vi "sweep over IDs.vi"() -> ()   [LabVIEW 2021, in "uCanDriver.lvlib" / "uCAN.lvclass"]
uses:
  uCAN.lvclass
  typedefs/bitrates.ctl
  typedefs/frame.ctl
panel:
  out "current ID":u32 format="%.0x"
  in  "Delay":i16
  in  "Stop":u32 format="%.0x"
  in  "Start":u32 format="%.0x"
  in  "Trace length":u64=100
  out "Table Control":string[][](table)
  in  "New Frame":T1 {"Data" format="%.0x"}
  in  "Bitrates":T2=enum."500 kbit/s"
  in  "COM port":refnum<visa-resource-name>="COM9"
  in  "stop":bool
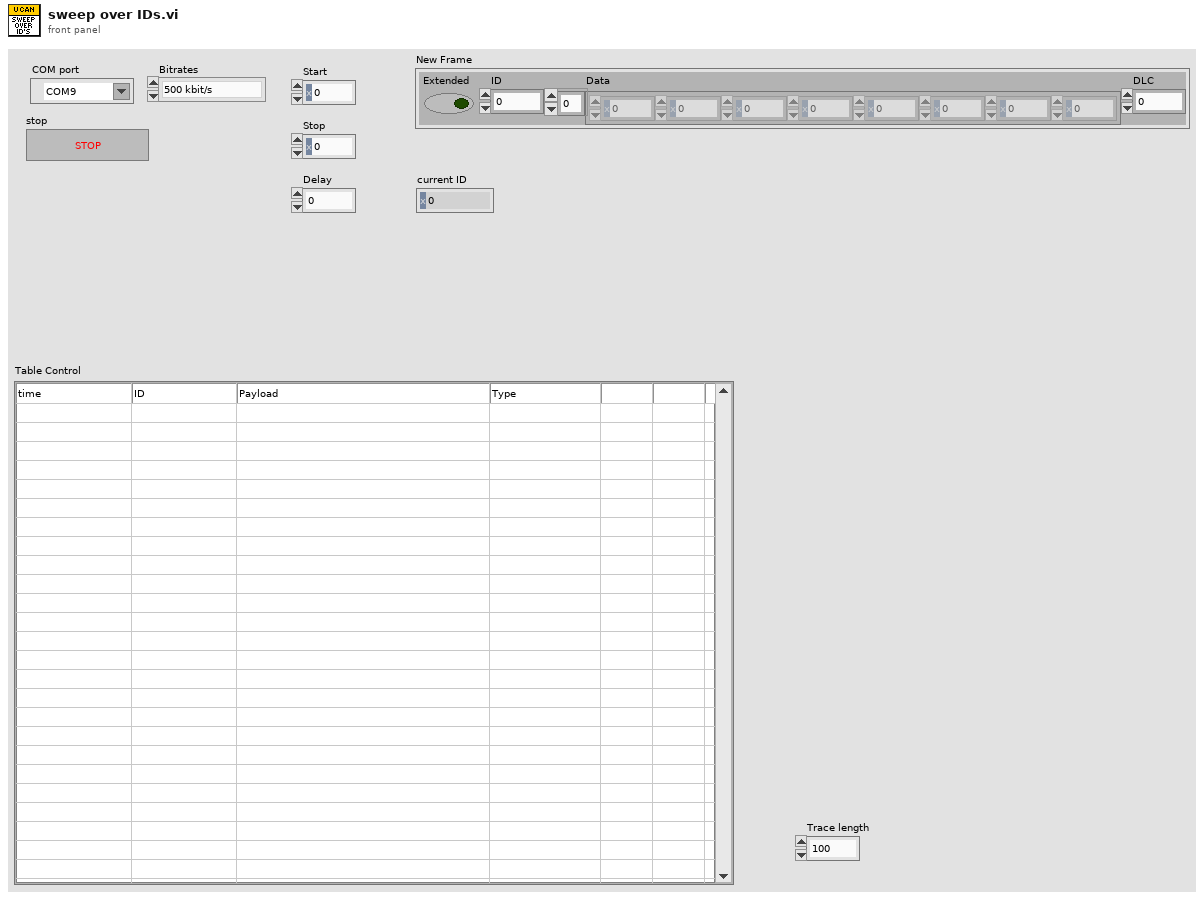
[diagram p1: front panel]
types:
  T1 = typedef "uCanDriver.lvlib/uCAN.lvclass/frame.ctl" = cluster{"Extended":bool, "ID":u32, "Data":u8[], "DLC":u8}
  T2 = typedef "uCanDriver.lvlib/uCAN.lvclass/bitrates.ctl" = enum16{"100 kbit/s", "125 kbit/s", "250 kbit/s", "500 kbit/s", "800 kbit/s", "1 Mbit/s"}
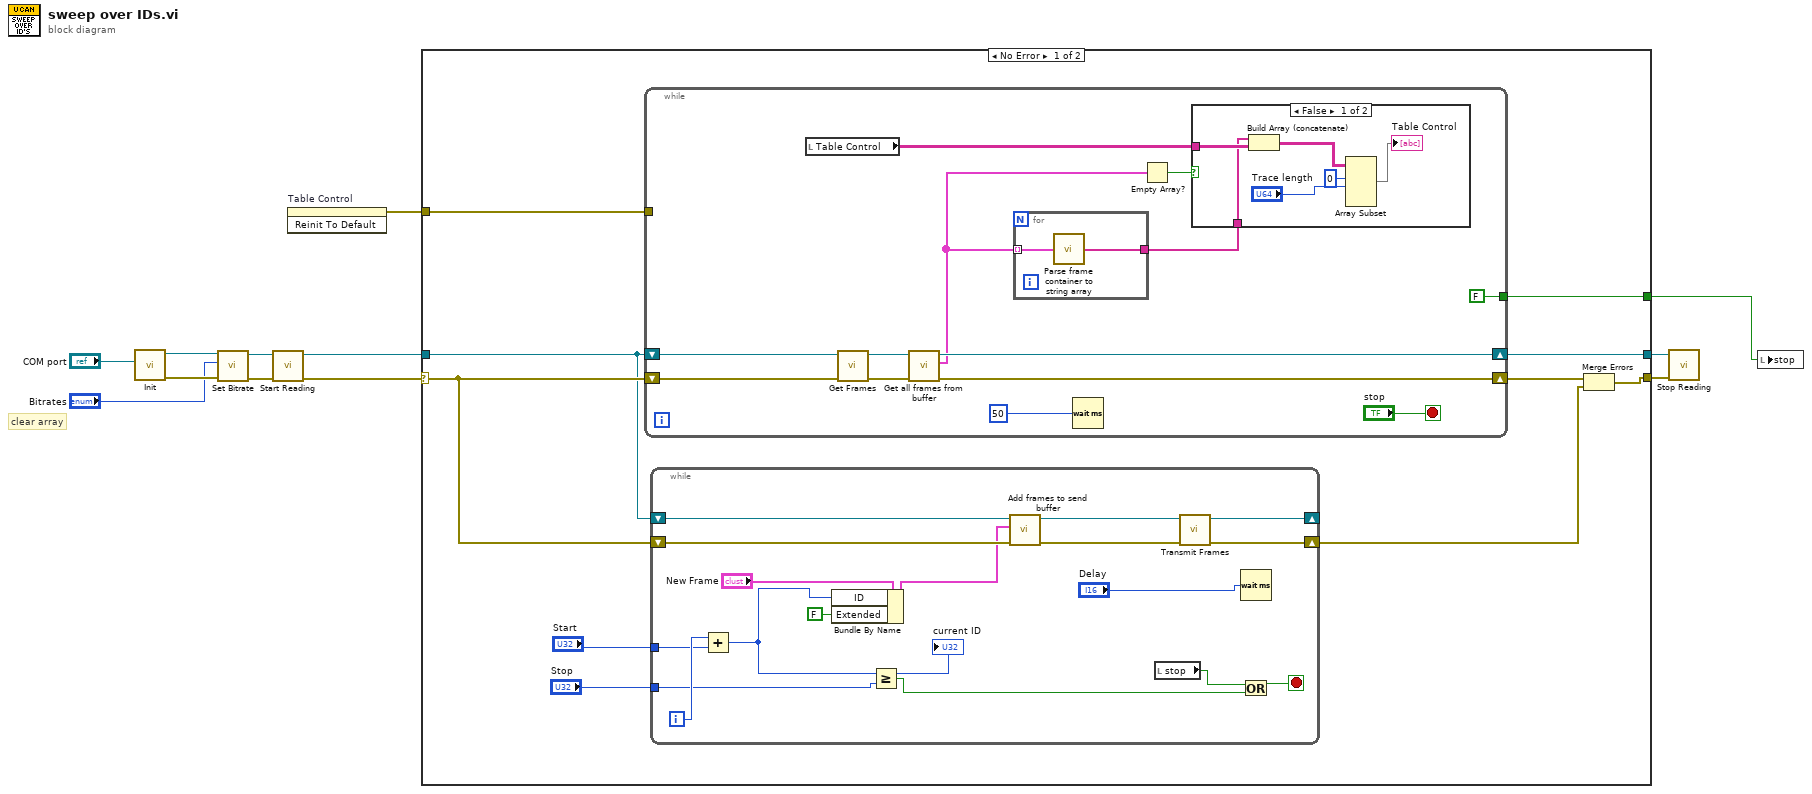
[diagram p0: block diagram]
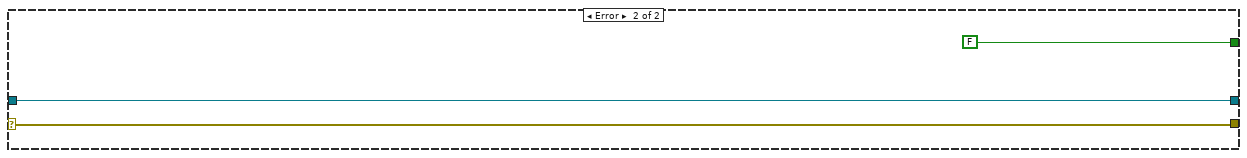
[diagram p3: hidden frame]
diagram:
  # "clear array"
  n1 = call "Init.vi"("COM port"="COM port") -> ("error out"=w10:errorcluster, "uCAN out"=w11:refnum<class "uCAN.lvclass">)  [unwired: 9 in]
  n2 = call "Set Bitrate.vi"("error in (no error)"=w10, "Bitrates"="Bitrates", "uCAN in"=w11) -> ("error out"=w6:errorcluster, "uCAN out"=w4:refnum<class "uCAN.lvclass">)  [unwired: 7 in]
  n3 = call "Start Reading.vi"("error in (no error)"=w6, "uCAN in"=w4) -> ("error out"=w5:errorcluster, "uCAN out"=w3:refnum<class "uCAN.lvclass">)  [unwired: 8 in]
  n4 = invoke on="Table Control" class="Tbl (strict)" method="Reinit To Default"() -> (error out=w2:errorcluster)  [unwired: 3 in, 2 out]
  n5 = case shown="No Error" w5 {
    selector: w5 -> [w18 w63]
    tunnel: [w22 w62] -> w8
    tunnel: [w20 w63] -> w7
    tunnel: w3 -> [w17 w62]
    tunnel: w2 -> [w16 _]
    tunnel: [w15 FALSE ("stop")] -> w1
    frame No Error {
      n6 = while {
        shift-right: [w31] -> w22
        shift-left: w17 -> [w35]
        shift-right: [w30] -> w21
        shift-left: w18 -> [w34]
        tunnel: w16 -> [_]
        tunnel: [FALSE ("stop")] -> w15
        stop <- "stop" stop-if-true
        n7 = local read "Table Control"() -> (w27:string[][])
        n8 = call "Get Frames.vi"("error in (no error)"=w34, "uCAN in"=w35) -> ("error out"=w33:errorcluster, "uCAN out"=w32:refnum<class "uCAN.lvclass">)  [unwired: 7 in, 1 out]
        n9 = call "Get all frames from buffer.vi"("error in (no error)"=w33, "uCAN in"=w32) -> ("error out"=w30:errorcluster, "Received Frames Array"=w23:T1[], "uCAN out"=w31:refnum<class "uCAN.lvclass">)  [unwired: 7 in]
        n10 = for {
          tunnel: [w37] -> w24
          tunnel: w23 -> [w36] mode=indexing
          n11 = call "Parse frame container to string array.vi"("Frame"=w36) -> ("String array"=w37:string[])
        }
        n12 = Wait (ms)(milliseconds to wait=u32 50) -> ()  [unwired: 1 out]
        n13 = Empty Array?(array=w23) -> (empty?=w26:bool)
        n14 = case shown="False" w26 {
          tunnel: w27 -> [w43 _]
          tunnel: w24 -> [w42 _]
          frame False {
            n15 = Build Array (concatenate)(w42, w43) -> (w39:string[][])
            n16 = Array Subset(array=w39, index (row)=0 ("index"), length (row)="Trace length") -> (→"Table Control":string[][])  [unwired: 2 in]
          }
          frame True {
          }
        }
      }
      n17 = while {
        shift-right: [w55] -> _
        shift-left: w17 -> [w60]
        shift-right: [w57] -> w19
        shift-left: w18 -> [w59]
        tunnel: "Start" -> [w49]
        tunnel: "Stop" -> [w46]
        i -> [w51]
        stop <- w48 stop-if-true
        n18 = Add(x=w51, y=w49) -> (x+y=w47:u32)
        "current ID" <- w47
        n19 = Bundle By Name(cluster="New Frame", "ID"=w47, "Extended"=FALSE) -> (w52:T1)
        n20 = Greater Or Equal?(x=w47, y=w46) -> (x >= y?=w45:bool)
        n21 = call "Add frames to send buffer.vi"("error in (no error)"=w59, "New Frame"=w52, "uCAN in"=w60) -> ("error out"=w58:errorcluster, "uCAN out"=w56:refnum<class "uCAN.lvclass">)  [unwired: 7 in]
        n22 = local read "stop"() -> (w54:bool)
        n23 = call "Transmit Frames.vi"("error in (no error)"=w58, "uCAN in"=w56) -> ("error out"=w57:errorcluster, "uCAN out"=w55:refnum<class "uCAN.lvclass">)  [unwired: 8 in]
        n24 = Wait (ms)(milliseconds to wait="Delay") -> ()  [unwired: 1 out]
        n25 = Or(x=w54, y=w45) -> (x .or. y?=w48:bool)
      }
      n26 = Merge Errors(w21, w19) -> (w20:errorcluster)
    }
    frame Error {
    }
  }
  n27 = call "Stop Reading.vi"("error in (no error)"=w7, "uCAN in"=w8) -> ()  [unwired: 8 in, 2 out]
  n28 = local write "stop"(w1) -> ()
